vi "Conv_Feet_Meters.vi"(10 "Feet":dbl) -> (2 "Meters":dbl)   [LabVIEW 2019, in "Trajectory_Library.lvlib"]
doc: "Convert Feet to Meters"
uses:
  Trajectory_Library.lvlib
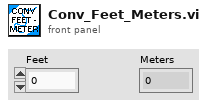
[diagram p1: front panel]
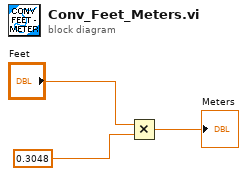
[diagram p0: block diagram]
diagram:
  n1 = Multiply(x="Feet", y=0.3048) -> (x*y=→"Meters":dbl)
